vi "Picture Coord to Row.vi"(9 "Row Height":i32, 10 "Coords":T1, 11 "Picture in":refnum<vi>) -> (2 "Row Index":i32, 3 "Clicked in canvas":bool)   [LabVIEW 2025]
uses:
  <vilib>/Utility/miscctls.llb/LVPoint32TypeDef.ctl
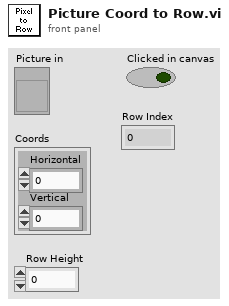
[diagram p1: front panel]
types:
  T1 = typedef "LVPoint32TypeDef.ctl" = cluster{"Horizontal":i32, "Vertical":i32}
  T2 = typedef "LVPointTypeDef.ctl" = cluster{"Horizontal":i16, "Vertical":i16}
  T3 = typedef "LVPositionTypeDef.ctl" = cluster{"Left":i32, "Top":i32}
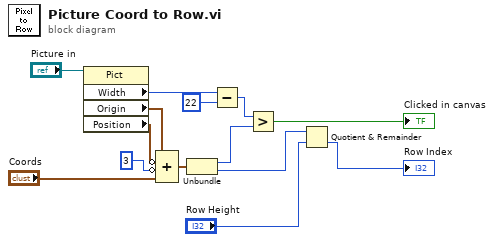
[diagram p0: block diagram]
diagram:
  n1 = property on="Property Node" class="Pict"(reference="Picture in") -> ("Width"=w9:u32, "Origin"=w6:T2, "Position"=w5:T3)  [unwired: 1 in, 2 out]
  n2 = Compound Arithmetic op=ADD(w6, invert w5, invert 3, "Coords") -> (w2:T3)
  n3 = Unbundle(w2) -> ("Left"=w8:i32, "Top"=w7:i32)
  n4 = Subtract(x=w9, y=u32 22) -> (x-y=w11:u32)
  n5 = Greater?(x=w11, y=w8) -> (0:→"Clicked in canvas":bool)
  n6 = Quotient & Remainder(x=w7, y="Row Height") -> (floor(x/y)=→"Row Index":i32)  [unwired: 1 out]
